vi "rx_ceEq.vi"(2 "preamble":cdb[](array[numeric])=[-0.7071067811865475+0.7071067811865476i, 0.7071067811865476+0.7071067811865475i, 0.7071067811865474-0.7071067811865477i, 0.7071067811865476+0.7071067811865475i, -0.7071067811865475+0.7071067811865476i, -0.7071067811865477-0.7071067811865475i, 0.7071067811865476+0.7071067811865475i, -0.7071067811865477-0.7071067811865475i, -0.7071067811865475+0.7071067811865476i, 0.7071067811865476+0.7071067811865475i, 0.7071067811865474-0.7071067811865477i, 0.7071067811865476+0.7071067811865475i, -0.7071067811865475+0.7071067811865476i, -0.7071067811865477-0.7071067811865475i, 0.7071067811865476+0.7071067811865475i, -0.7071067811865477-0.7071067811865475i, -0.7071067811865475+0.7071067811865476i, 0.7071067811865476+0.7071067811865475i, 0.7071067811865474-0.7071067811865477i, 0.7071067811865476+0.7071067811865475i, -0.7071067811865475+0.7071067811865476i, -0.7071067811865477-0.7071067811865475i, 0.7071067811865476+0.7071067811865475i, -0.7071067811865477-0.7071067811865475i, -0.7071067811865475+0.7071067811865476i, 0.7071067811865476+0.7071067811865475i, 0.7071067811865474-0.7071067811865477i, 0.7071067811865476+0.7071067811865475i, -0.7071067811865475+0.7071067811865476i, -0.7071067811865477-0.7071067811865475i, 0.7071067811865476+0.7071067811865475i, -0.7071067811865477-0.7071067811865475i, -0.7071067811865475+0.7071067811865476i, 0.7071067811865476+0.7071067811865475i, 0.7071067811865474-0.7071067811865477i, 0.7071067811865476+0.7071067811865475i, -0.7071067811865475+0.7071067811865476i, -0.7071067811865477-0.7071067811865475i, 0.7071067811865476+0.7071067811865475i, -0.7071067811865477-0.7071067811865475i, -0.7071067811865475+0.7071067811865476i, 0.7071067811865476+0.7071067811865475i, 0.7071067811865474-0.7071067811865477i, 0.7071067811865476+0.7071067811865475i, -0.7071067811865475+0.7071067811865476i, -0.7071067811865477-0.7071067811865475i, 0.7071067811865476+0.7071067811865475i, -0.7071067811865477-0.7071067811865475i, -0.7071067811865475+0.7071067811865476i, 0.7071067811865476+0.7071067811865475i, 0.7071067811865474-0.7071067811865477i, 0.7071067811865476+0.7071067811865475i, -0.7071067811865475+0.7071067811865476i, -0.7071067811865477-0.7071067811865475i, 0.7071067811865476+0.7071067811865475i, -0.7071067811865477-0.7071067811865475i, -0.7071067811865475+0.7071067811865476i, 0.7071067811865476+0.7071067811865475i, 0.7071067811865474-0.7071067811865477i, 0.7071067811865476+0.7071067811865475i, -0.7071067811865475+0.7071067811865476i, -0.7071067811865477-0.7071067811865475i, 0.7071067811865476+0.7071067811865475i, -0.7071067811865477-0.7071067811865475i], 3 "symbols":cdb[](array[numeric])) -> (0 "valid?":bool, 1 "eq symbols":cdb[](array[numeric]))   [LabVIEW 2014]
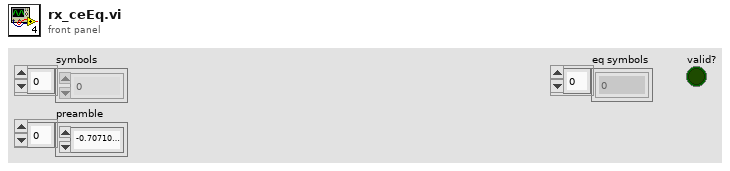
[diagram p1: front panel]
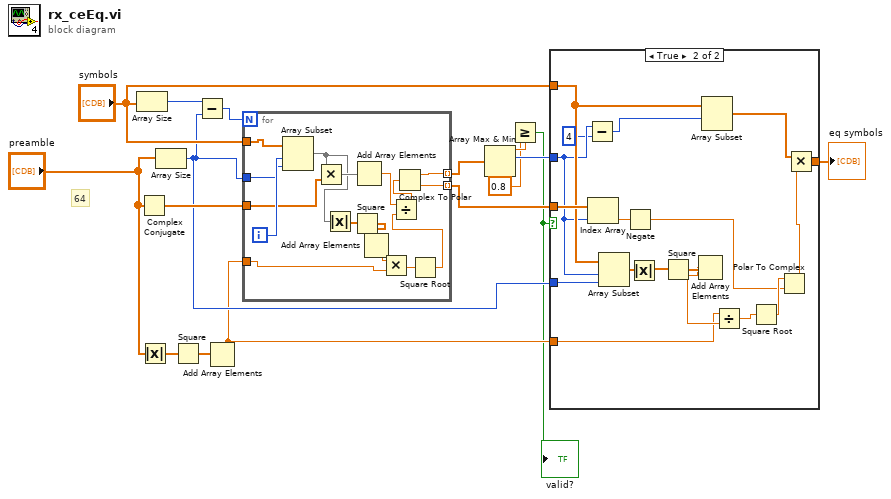
[diagram p0: block diagram]
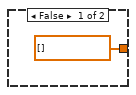
[diagram p2: hidden frame]
diagram:
  # "64"
  n1 = Array Size(array="symbols") -> (size(s)=w16:i32)
  n2 = Complex Conjugate(1:"preamble") -> (0:w14:cdb[])
  n3 = Absolute Value(x="preamble") -> (abs(x)=w10:dbl[])
  n4 = Array Size(array="preamble") -> (size(s)=w6:i32)
  n5 = Square(x=w10) -> (x^2=w9:dbl[])
  n6 = Subtract(x=w16, y=w6) -> (x-y=w15:i32)
  n7 = Add Array Elements(numeric array=w9) -> (sum=w4:dbl)
  n8 = for {
    N: w15 -> [_]
    tunnel: "symbols" -> [w32]
    tunnel: w14 -> [w29]
    tunnel: w6 -> [w30]
    tunnel: [w27] -> w13 mode=indexing
    tunnel: [w26] -> w12 mode=indexing
    tunnel: w4 -> [w21]
    i -> [w31]
    n9 = Array Subset(array=w32, index=w31, length=w30) -> (w25:cdb[])
    n10 = Multiply(x=w25, y=w29) -> (x*y=w28:cdb[])
    n11 = Absolute Value(x=w25) -> (abs(x)=w24:dbl[])
    n12 = Square(x=w24) -> (x^2=w23:dbl[])
    n13 = Add Array Elements(numeric array=w28) -> (sum=w20:cdb)
    n14 = Add Array Elements(numeric array=w23) -> (sum=w22:dbl)
    n15 = Multiply(x=w22, y=w21) -> (x*y=w19:dbl)
    n16 = Square Root(x=w19) -> (sqrt(x)=w18:dbl)
    n17 = Divide(x=w20, y=w18) -> (x/y=w17:cdb)
    n18 = Complex To Polar(r * e^(i*theta)=w17) -> (r=w27:dbl, theta=w26:dbl)
  }
  n19 = Array Max & Min(array=w13) -> (max value=w3:dbl, max index (indices)=w7:i32)  [unwired: 2 out]
  n20 = Greater Or Equal?(x=w3, y=0.8) -> (x >= y?=w1:bool)
  "valid?" <- w1
  n21 = case shown="True" w1 {
    tunnel: w12 -> [_ w51]
    tunnel: "symbols" -> [_ w49]
    tunnel: w7 -> [_ w36]
    tunnel: w6 -> [_ w37]
    tunnel: [cdb[] [] w39] -> w5
    tunnel: w4 -> [_ w38]
    frame False {
    }
    frame True {
      n22 = Subtract(x=w36, y=4) -> (x-y=w34:i32)
      n23 = Index Array(array=w51, index=w36) -> (element=w50:dbl)
      n24 = Array Subset(array=w49, index=w36, length=w37) -> (w48:cdb[])
      n25 = Negate(x=w50) -> (-x=w42:dbl)
      n26 = Absolute Value(x=w48) -> (abs(x)=w47:dbl[])
      n27 = Square(x=w47) -> (x^2=w46:dbl[])
      n28 = Add Array Elements(numeric array=w46) -> (sum=w45:dbl)
      n29 = Array Subset(array=w49, index=w34) -> (w40:cdb[])  [unwired: 1 in]
      n30 = Divide(x=w38, y=w45) -> (x/y=w44:dbl)
      n31 = Square Root(x=w44) -> (sqrt(x)=w43:dbl)
      n32 = Polar To Complex(1:w42, 2:w43) -> (0:w41:cdb)
      n33 = Multiply(x=w40, y=w41) -> (x*y=w39:cdb[])
    }
  }
  "eq symbols" <- w5
